vi "Get Obj Z Pos.vi"(0 "Notifier Name In":string, 11 "Error In":errorcluster) -> (4 "Notifier Name Out":string, 8 "Obj Z Pos":dbl, 15 "Error Out":errorcluster)   [LabVIEW 2020]
uses:
  Microscopes Type Defs/Microscope Notifier.ctl
  Microscopes Type Defs/Microscope Actions.ctl
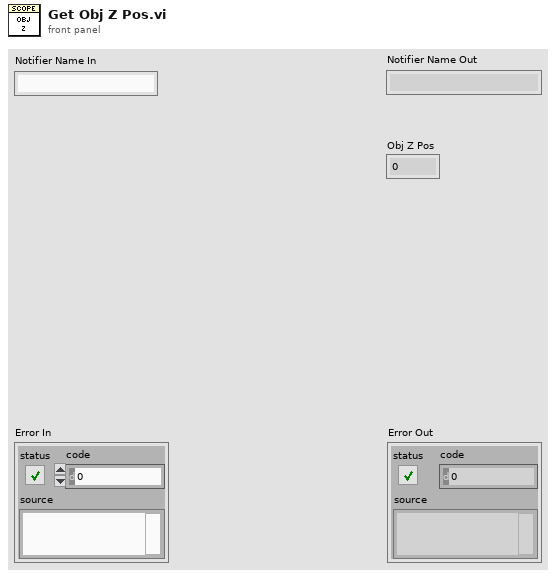
[diagram p1: front panel]
types:
  T1 = typedef "Microscope Notifier.ctl" = cluster{"Actions":T2, "Action Done":bool, "Objective Index":u8, "Objective Z Position (um)":dbl, "Lamp Index":u8, "Lamp State":bool, "Output Port":u8, "Shutter Index":u8, "Shutter State":bool, "Dichroic Wheel Position":u8, "Parameter":string, "Parameter Value":string, "Base Locked?":bool, "Obj Speed":u32, "Obj Acceleration":u32, "Obj Deceleration":u32, "Lamp Power (%)":dbl, "Dichroic Wheel Index":u8}
  T2 = typedef "Microscope Actions.ctl" = enum16{"Do Nothing", "Lock Base", "Lock Focus Knob", "Get Objective Index", "Get Objective Z Position", "Get Lamp State", "Get Lamp Power", "Get Output Port", "Get Shutter State", "Get Dichroic Wheel Position", "Set Lamp Index", "Set Shutter Index", "Set Objective Z Position", "Set Lamp State", "Set Lamp Power", "Set Output Port", "Set Shutter State", "Set Dichroic Wheel Position", "Set Objective", "Abort Move", "Set Parameter", "Get Parameter", "Quit"}
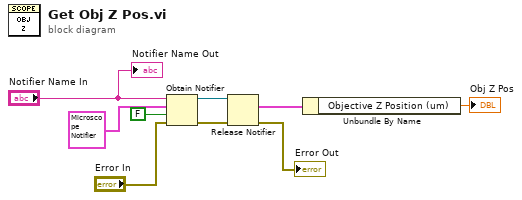
[diagram p0: block diagram]
diagram:
  n1 = Obtain Notifier(name (unnamed)="Notifier Name In", notification data type=T1 {"Actions"=enum."Get Objective Index", "Action Done"=FALSE, "Objective Index"=0, "Objective Z Position (um)"=0.0, "Lamp Index"=0, "Lamp State"=FALSE, "Output Port"=0, "Shutter Index"=0, "Shutter State"=FALSE, "Dichroic Wheel Position"=0, "Parameter"="", "Parameter Value"="", "Base Locked?"=FALSE, "Obj Speed"=0, "Obj Acceleration"=0, "Obj Deceleration"=0, "Lamp Power (%)"=0.0, "Dichroic Wheel Index"=0} ("Microscope Notifier"), create if not found? (T)=FALSE, error in (no error)="Error In") -> (notifier out=w4:refnum<notifier>, error out=w3:errorcluster)  [unwired: 1 out]
  n2 = Release Notifier(notifier=w4, error in (no error)=w3) -> (last notification=w2:T1, error out=→"Error Out":errorcluster)  [unwired: 1 in, 1 out]
  n3 = Unbundle By Name(w2) -> ("Objective Z Position (um)"=→"Obj Z Pos":dbl)
  "Notifier Name Out" <- "Notifier Name In"
